vi "读取本地版本号.vi"() -> (6 "版本号":string, 7 "版本路径":path, 8 "错误?":bool=TRUE)   [LabVIEW 2017]
uses:
  <vilib>/Utility/config.llb/Read Key (String).vi
  <vilib>/Utility/config.llb/NI_LVConfig.lvlib
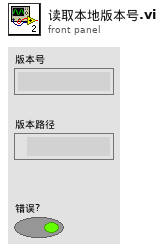
[diagram p1: front panel]
types:
  T1 = typedef "NI_LVConfig.lvlib/Config Data RefNum.ctl" = refnum<k1>
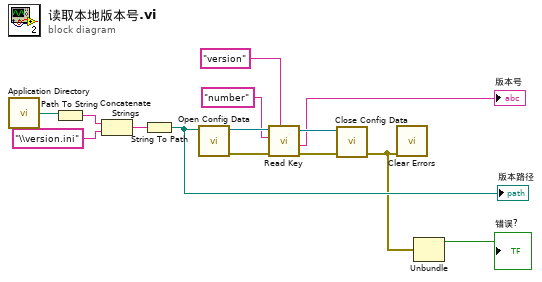
[diagram p0: block diagram]
diagram:
  n1 = call <vilib>:"Application Directory.vi"() -> ("Application Directory"=w13:path)
  n2 = Path To String(path=w13) -> (string=w12:string)
  n3 = Concatenate Strings(w12, "\\version.ini") -> (w11:string)
  n4 = String To Path(string=w11) -> (path=w5:path)
  "版本路径" <- w5
  n5 = call <vilib>:"Open Config Data.vi"("configuration file path"=w5) -> ("error out"=w6:errorcluster, "refnum"=w10:T1)  [unwired: 8 in, 1 out]
  n6 = call-poly <vilib>:"Read Key.vi"("section"="version", "error in (no error)"=w6, "key"="number", "refnum"=w10) -> ("error out"=w3:errorcluster, "value"=→"版本号":string, "refnum out"=w7:T1)  [unwired: 4 in, 1 out]
  n7 = call <vilib>:"Close Config Data.vi"("error in (no error)"=w3, "refnum"=w7) -> ("error out"=w2:errorcluster)  [unwired: 8 in, 1 out]
  n8 = call <vilib>:"Clear Errors.vi"("error in (no error)"=w2) -> ()  [unwired: 5 in, 2 out]
  n9 = Unbundle(w2) -> ("status"=→"错误?":bool)  [unwired: 2 out]
